vi "configuration_si.vi"() -> (3 "configuration_si":cluster{"chunk":u64}={"chunk"=1024})   [LabVIEW 2023]
panel:
  in  "configuration_si":cluster{"chunk":u64}={"chunk"=1024}
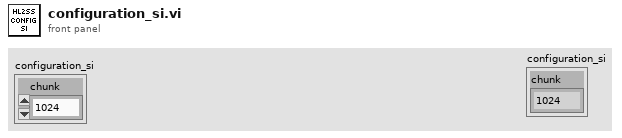
[diagram p1: front panel]
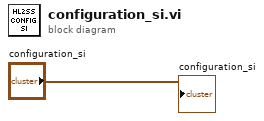
[diagram p0: block diagram]
diagram:
  "configuration_si" <- "configuration_si"
